vi "Global Mapper G.vi"(10 "Trail off/on":bool, 11 "GIC Input":T1={"     Use ?\nOff       On"=[FALSE, TRUE, FALSE, TRUE], "Mode:"=FALSE, "WP Data"="", "Hokuyo Port"="COM7", "Prop  Port"="COM6", "Compass Port"="", "GPS Port"="", "Num of WPs"=0, "WP Lats and Longs"={"WP Lats"=[], "WP Longs"=[]}, "Obst Lats and Longs"={"Obst Lats"=[], "Obst Longs"=[]}, "Parameters"=[], "GPS Data"=[], "Compass"=0.0, "LMS Vector"=[], "Vision Vector"=[], "Direction Cmd"=0.0, "Speed Cmd"=0.0, "WP Vector"=[], "WP Number"=0, "Extra"=0, "SW Map"=[], "Path Cluster"={"Path x node"=[], "Path y node"=[]}, "Sim Course"=[]} {"Obst Lats and Longs"."Obst Longs" format="%#_8g"; "Obst Lats and Longs"."Obst Lats" format="%#_8g"}) -> (0 "picture out":picture)   [LabVIEW 2014]
panel:
  in  "picture in":picture
  # "Global Mapper G"
  # "Inputs:"
  # "Output:"
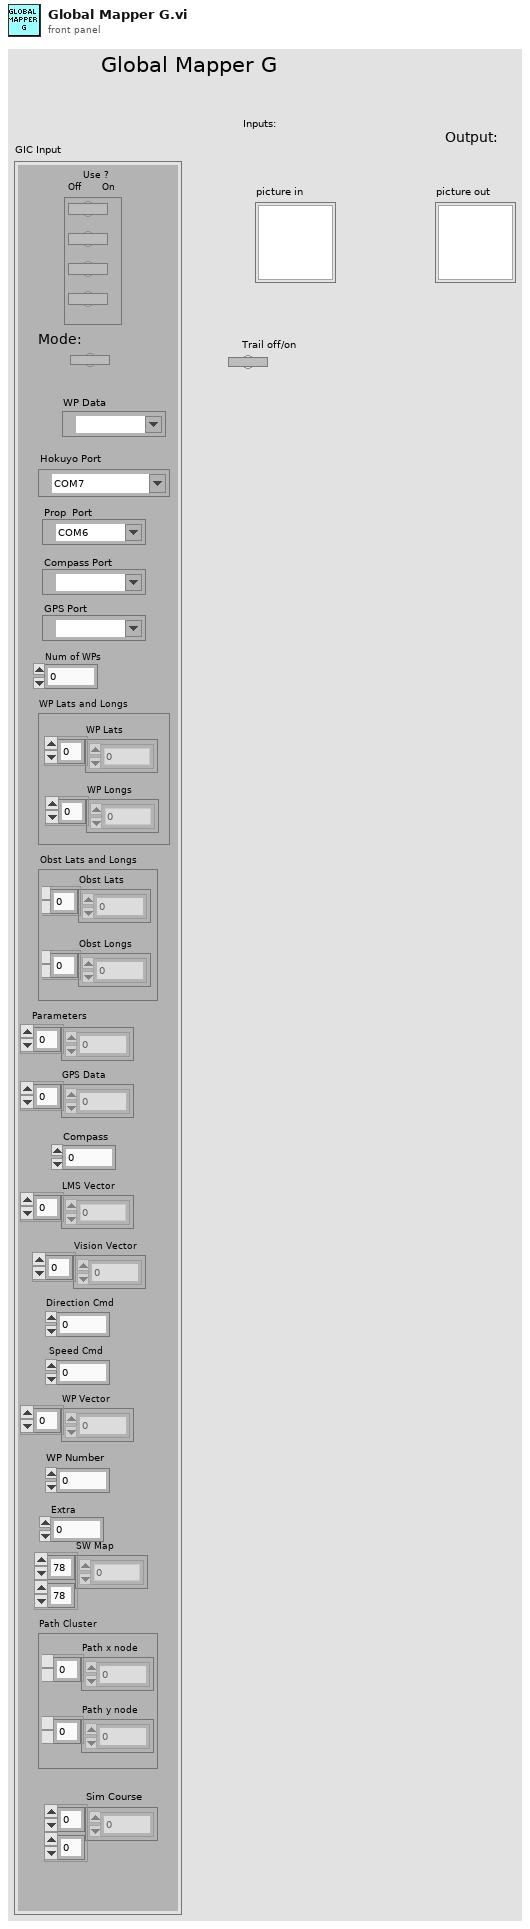
[diagram p1: front panel]
types:
  T1 = cluster{"     Use ?\nOff       On":bool[], "Mode:":bool, "WP Data":refnum<visa-resource-name>, "Hokuyo Port":refnum<visa-resource-name>, "Prop  Port":refnum<visa-resource-name>, "Compass Port":refnum<visa-resource-name>, "GPS Port":refnum<visa-resource-name>, "Num of WPs":i16, "WP Lats and Longs":cluster{"WP Lats":dbl[], "WP Longs":dbl[]}, "Obst Lats and Longs":cluster{"Obst Lats":dbl[], "Obst Longs":dbl[]}, "Parameters":dbl[], "GPS Data":dbl[], "Compass":dbl, "LMS Vector":dbl[], "Vision Vector":dbl[], "Direction Cmd":dbl, "Speed Cmd":dbl, "WP Vector":dbl[], "WP Number":i32, "Extra":i16, "SW Map":i32[][], "Path Cluster":cluster{"Path x node":dbl[], "Path y node":dbl[]}, "Sim Course":i8[][]}
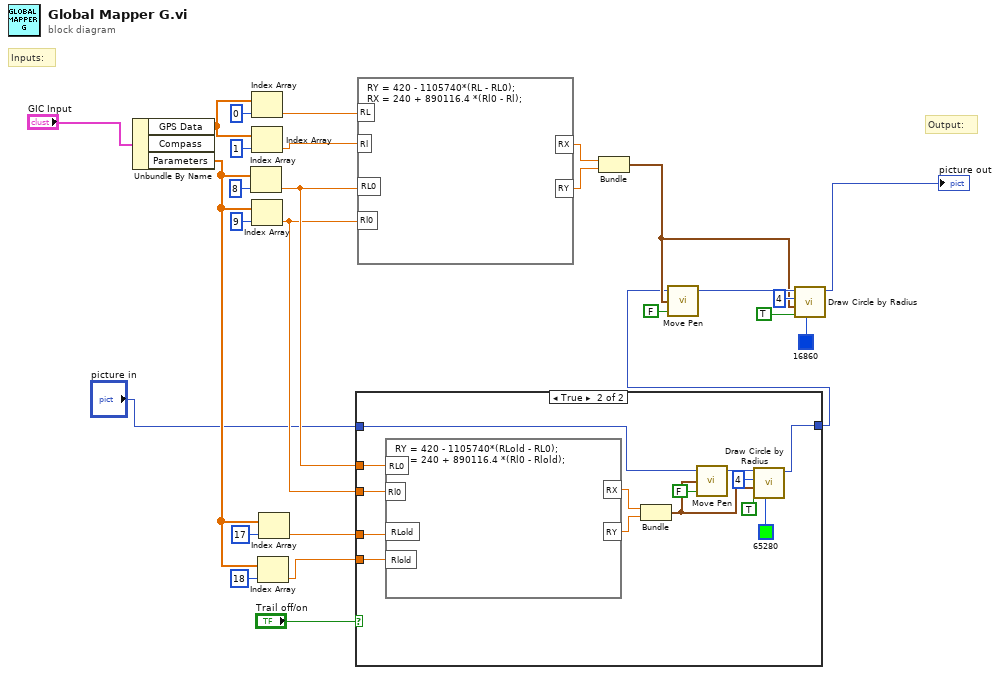
[diagram p0: block diagram]
diagram:
  # "Output:"
  # "Inputs:"
  n1 = Unbundle By Name("GIC Input") -> ("GPS Data"=w24:dbl[], "Parameters"=w9:dbl[])  [unwired: 1 out]
  n2 = Index Array(array=w9, index=8) -> (element=w7:dbl)
  n3 = Index Array(array=w24, index=0) -> (element=w26:dbl)
  n4 = Index Array(array=w24, index=1) -> (element=w22:dbl)
  n5 = Index Array(array=w9, index=9) -> (element=w6:dbl)
  n6 = Index Array(array=w9, index=18) -> (element=w4:dbl)
  n7 = Index Array(array=w9, index=17) -> (element=w5:dbl)
  n8 = case shown="True" "Trail off/on" {
    tunnel: w7 -> [_ w42]
    tunnel: w6 -> [_ w41]
    tunnel: w5 -> [_ w40]
    tunnel: w4 -> [_ w39]
    tunnel: [w28 w35] -> w2
    tunnel: "picture in" -> [w28 w29]
    frame False {
    }
    frame True {
      n9 = formula code="RY = 420 - 1105740*(RLold - RL0);\nRX = 240 + 890116.4 *(Rl0 - Rlold);"("RL0"=w42, "Rl0"=w41, "RLold"=w40, "Rlold"=w39) -> ("RX"=w38:dbl, "RY"=w37:dbl)
      n10 = Bundle("RX"=w38, "RY"=w37) -> (w34:cluster{"RX":dbl, "RY":dbl})  [unwired: 1 in]
      n11 = call <vilib>:"Move Pen.vi"("absolute coordinates?(T)"=FALSE, "new position"=w34, "picture"=w29) -> ("new picture"=w36:picture)  [unwired: 2 in]
      n12 = call <vilib>:"Draw Circle by Radius.vi"("color(black)"=u32 65280, "fill?(F)"=TRUE, "pixel center"=w34, "radius"=i16 4, "picture"=w36) -> ("new picture"=w35:picture)  [unwired: 6 in]
    }
  }
  n13 = formula code="RY = 420 - 1105740*(RL - RL0);\nRX = 240 + 890116.4 *(Rl0 - Rl);"("RL"=w26, "Rl"=w22, "RL0"=w7, "Rl0"=w6) -> ("RY"=w17:dbl, "RX"=w18:dbl)
  n14 = Bundle("RX"=w18, "RY"=w17) -> (w12:cluster{"RX":dbl, "RY":dbl})  [unwired: 1 in]
  n15 = call <vilib>:"Move Pen.vi"("absolute coordinates?(T)"=FALSE, "new position"=w12, "picture"=w2) -> ("new picture"=w19:picture)  [unwired: 2 in]
  n16 = call <vilib>:"Draw Circle by Radius.vi"("color(black)"=u32 16860, "fill?(F)"=TRUE, "pixel center"=w12, "radius"=i16 4, "picture"=w19) -> ("new picture"=→"picture out":picture)  [unwired: 6 in]
